vi "SetTemperature.vi"(0 "reference in":refnum<class "HeatingSystem.lvclass">, 2 "RoomName":string, 3 "TemperatureValue":dbl, 5 "Error In":errorcluster) -> (14 "reference out":refnum<class "HeatingSystem.lvclass">, 19 "Error Out":errorcluster)   [LabVIEW 2024, in "HeatingSystem.lvclass"]
doc: "Takes RoomName and desired Temperature value and sets temperature of all the heating systems in the given room."
uses:
  HeatingSystem.lvclass
  House/Room_class/Room.lvclass
  Devices/Air Conditioner_class/Air Conditioner.lvclass
panel:
  # "Connector Pane"
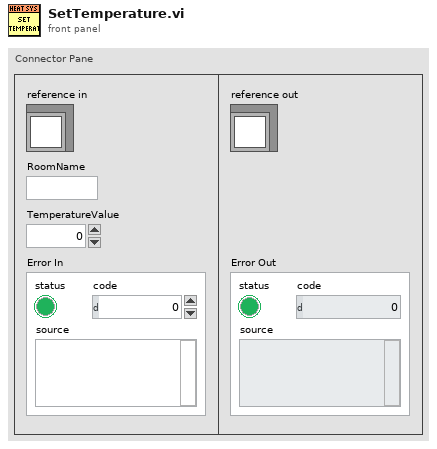
[diagram p1: front panel]
types:
  T1 = typedef "HeatingSystem.lvclass/ObjectAttributes.ctl" = cluster{"Rooms":T2}
  T2 = typedef "Rooms Map.ctl" = map{string, refnum<class "Room.lvclass">}
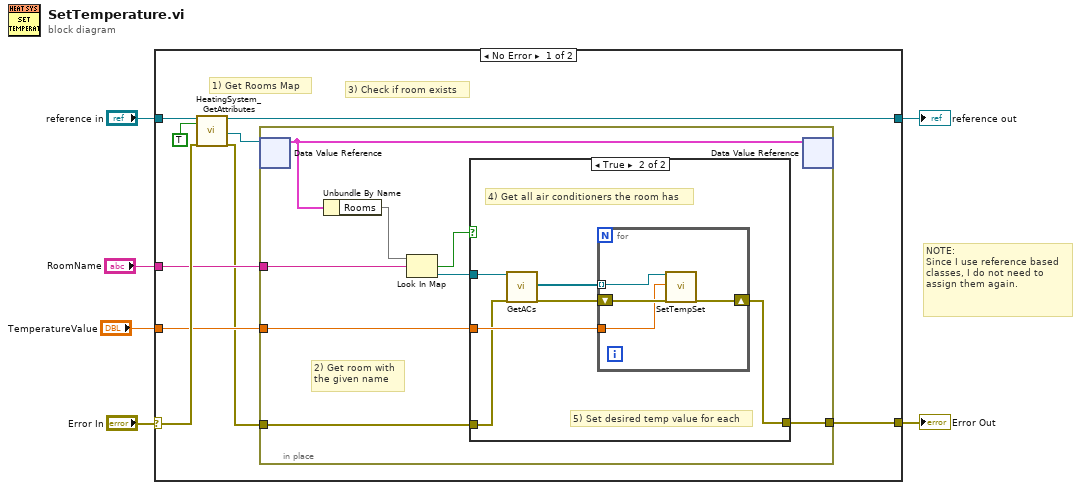
[diagram p0: block diagram]
diagram:
  # "NOTE:\nSince I use reference based classes, I do not need to\nassign them again."
  n1 = case shown="No Error" "Error In" {
    selector: "Error In" -> [w14 w36]
    tunnel: [w7 w36] -> w5
    tunnel: [w13 w35] -> w3
    tunnel: "reference in" -> [w15 w35]
    tunnel: "RoomName" -> [w10 _]
    tunnel: "TemperatureValue" -> [w9 _]
    frame No Error {
      # "3) Check if room exists"
      # "1) Get Rooms Map"
      n2 = call "HeatingSystem_GetAttributes.vi"("reference in"=w15, "OnlyGetDvrReference(False)"=TRUE, "Error In"=w14) -> ("reference out"=w13:refnum<class "HeatingSystem.lvclass">, "DataRef"=w12:refnum<data-value>, "Error Out"=w8:errorcluster)  [unwired: 13 in, 1 out]
      n3 = in-place {
        in-place-border: w10 -> [w21]
        in-place-border: w9 -> [w18]
        in-place-border: w8 -> [w17]
        in-place-border: [w16] -> w7
        # "2) Get room with\nthe given name"
        n4 = in-place-dvr #1(w12) -> (w23:T1)  [unwired: 1 out]
        n5 = Unbundle By Name(w23) -> ("Rooms"=w22:T2)
        n6 = Look In Map(map=w22, key=w21) -> (key not found?=w20:bool, value=w19:refnum<class "Room.lvclass">)  [unwired: 1 in]
        n7 = case shown="True" w20 {
          tunnel: w19 -> [_ w30]
          tunnel: w18 -> [_ w27]
          tunnel: w17 -> [w24 w26]
          tunnel: [w24 w25] -> w16
          frame False {
          }
          frame True {
            # "5) Set desired temp value for each"
            # "4) Get all air conditioners the room has"
            n8 = call-dynamic "GetACs.vi"("reference in"=w30, "Error In"=w26) -> ("ACs"=w28:refnum<class "Air Conditioner.lvclass">[], "Error Out"=w29:errorcluster)  [unwired: 15 in, 1 out]
            n9 = for {
              tunnel: w28 -> [w33] mode=indexing
              tunnel: w27 -> [w32]
              shift-right: [w31] -> w25
              shift-left: w29 -> [w34]
              n10 = call-dynamic "SetTempSet.vi"("reference in"=w33, "TempSet"=w32, "Error In"=w34) -> ("Error Out"=w31:errorcluster)  [unwired: 15 in, 1 out]
            }
          }
        }
        n11 = in-place-dvr #1(w23) -> ()  [unwired: 2 out]
      }
    }
    frame Error {
    }
  }
  "Error Out" <- w5
  "reference out" <- w3
